vi "FPGAmain_5782_amtest.vi"() -> ()   [LabVIEW 2013]
uses:
  FPGA/DataMode.ctl
  FPGA/Input_5782/5782_states.ctl
  <vilib>/Platform/TimedLoop/XDataNode/timing_clust.ctl
  <vilib>/Platform/TimedLoop/XDataNode/nitl_modes.ctl
  <vilib>/Platform/TimedLoop/XDataNode/wakeup.ctl
  <vilib>/rvi/Emulation/niFpgaSctlEmulationGetInTimedLoop.vi
  <vilib>/rvi/Emulation/niFpgaEmulationReportErrorSimple.vi
  <vilib>/rvi/Emulation/niFpgaGetClockAttributes.vi
  <vilib>/rvi/eio/common/nirviEmuTemplateMethod_errors.vi
  <vilib>/rvi/Emulation/niFpgaCriticalErrorInLSC.vi
  <vilib>/rvi/FIFO/Fifo_Resource/nirvififoEmulationReadFpgaImpl.vi
  <vilib>/rvi/DataTransferAndStorage/Container/Common/niFpgaContainerGetUniqueNameForEmu.vi
  <vilib>/rvi/interface/RandomDataEmulation/nirviRandomDataFPGAFIFO.vi
  <vilib>/rvi/interface/RandomDataEmulation/niFpgaRandomDataHandleErrors.vi
  <vilib>/rvi/DataTransferAndStorage/Register/Emulation/niFpgaRegisterEmulationFpgaImpl.vi
  <instcachedir>/0/niFpgaRegisterEmulationFpgaImpl_DCF4BC0110594B98B44A971D60CEEC4D.lvgen/niFpgaRegisterEmulationFpgaImpl_DCF4BC0110594B98B44A971D60CEEC4D_003.vi
  <vilib>/rvi/FIFO/Fifo_Resource/nirvififoEmulationWriteFpgaImpl.vi
  <vilib>/Platform/TimedLoop/XDataNode/XDataNode.xnode
  <vilib>/eio/EIONode/EIONode.xnode
  <vilib>/rvi/DataTransferAndStorage/Container/XNode/niFpgaContainer.xnode
  <vilib>/rvi/FIFO/Fifo_Resource/nirvififoEmulationRead.vi
  <vilib>/rvi/interface/RandomDataEmulation/nirviRandomDataFpgaReadWriteTemplate.vi
  <vilib>/rvi/DataTransferAndStorage/Register/Emulation/niFpgaRegisterEmulation.vi
  <vilib>/rvi/FIFO/Fifo_Resource/nirvififoEmulationWrite.vi
  <vilib>/Platform/TimedLoop/XDataNode/XDNodeRunTimeDep.lvlib
panel:
  in  "b_am":fxp<+/-,16,2>
  in  "a_am":fxp<+/-,16,2>
  in  "AM phase":fxp<+,64,64>
  in  "DC offset chan 0":fxp<+/-,16,16>
  in  "DC offset chan 1":fxp<+/-,16,16>
  in  "delay phase":fxp<+,64,64>
  in  "User Command Commit":bool
  in  "User Command":u8
  out "User Command Idle":bool
  out "User Command Status":u8
  in  "User Data 0":u8
  in  "User Data 1":u8
  out "PLL Locked":bool
  out "User Error":bool
  out "Configured?":bool
  in  "Continuous":bool
  in  "trigger samples":u16=1
  in  "5782 record length":u16=4000 caption="Samples Per Trigger" min=1 step=1
  in  "Trigger Acquisition":bool
  out "IO Module\\Trigger Input":bool
  in  "quiet time":u16=4000
  in  "Downsample":fxp<+,8,8>=1.0
  in  "enable filter":bool
  in  "new coeffs":bool
  in  "FIR shift":i32
  in  "FIR coeffs":fxp<+/-,18,18>[](array[numeric])
  in  "Set downsample":bool
  in  "CIC Gain":fxp<+/-,32,1>=0.00390625 format="%#_32g"
  in  "Acquisition running":bool
  in  "Phase output":fxp<+,64,64>[](array[numeric])=[0.0, 0.0, 0.0, 0.0]
  in  "Simulated phase 5782":fxp<+,64,64>[](array[numeric])=[0.0, 0.0]
  in  "Mode":T1
  in  "Phase 5782":fxp<+,64,64>[](array[numeric])=[0.0, 0.0]
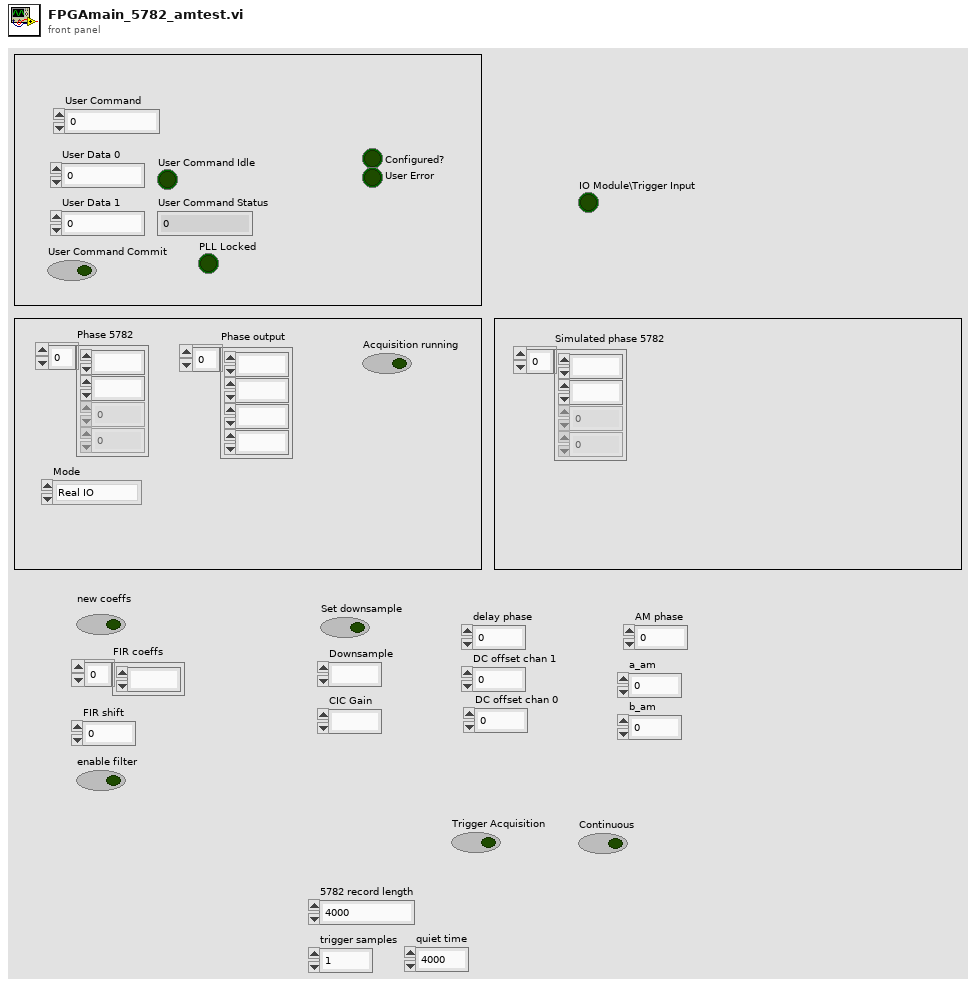
[diagram p1: front panel]
types:
  T1 = typedef "DataMode.ctl" = enum16{"Real IO", "Simulated"}
  T2 = typedef "5782_states.ctl" = enum8{"Wait for trigger", "Acquisition", "Send record length", "Quiet period"}
  T3 = typedef "XDNodeRunTimeDep.lvlib/timing_clust.ctl" = cluster{"Expected End [f-1]":u64, "Actual End [f-1]":u64, "Finished Late? [f-1]":bool, "Expected End [i-1]":u64, "Actual End [i-1]":u64, "Finished Late? [i-1]":bool, "Expected Start [i]":u64, "Actual Start [i]":u64, "Expected Start [f]":u64, "Actual Start [f]":u64, "Source Name":string, "Structure Name":string, "Period":i64, "Deadline":i64, "Offset":i64, "Start":i64, "Priority":i32, "Timeout":i32, "Mode":T4, "Wakeup Reason":T5, "Error":errorcluster, "Source Type":string, "Secondary Source Type":string, "Global End Time":u64, "Global Start Time":u64, "Frame Duration":u64, "Iteration Duration":u64, "Assigned CPU":i32, "I/O Scan Engine Mode":u32}
  T4 = typedef "XDNodeRunTimeDep.lvlib/nitl_modes.ctl" = enum32{"No Change", "Process missed periods, maintain original phase", "Discard missed periods, maintain original phase", "Process missed periods, ignore original phase", "Discard missed periods, ignore original phase"}
  T5 = typedef "XDNodeRunTimeDep.lvlib/wakeup.ctl" = enum32{"Normal", "Aborted", "Asynchronous wakeup", "Timing source error", "Timed loop error", "Timeout"}
  T6 = typedef "I16 array size 2.ctl" = i16[]
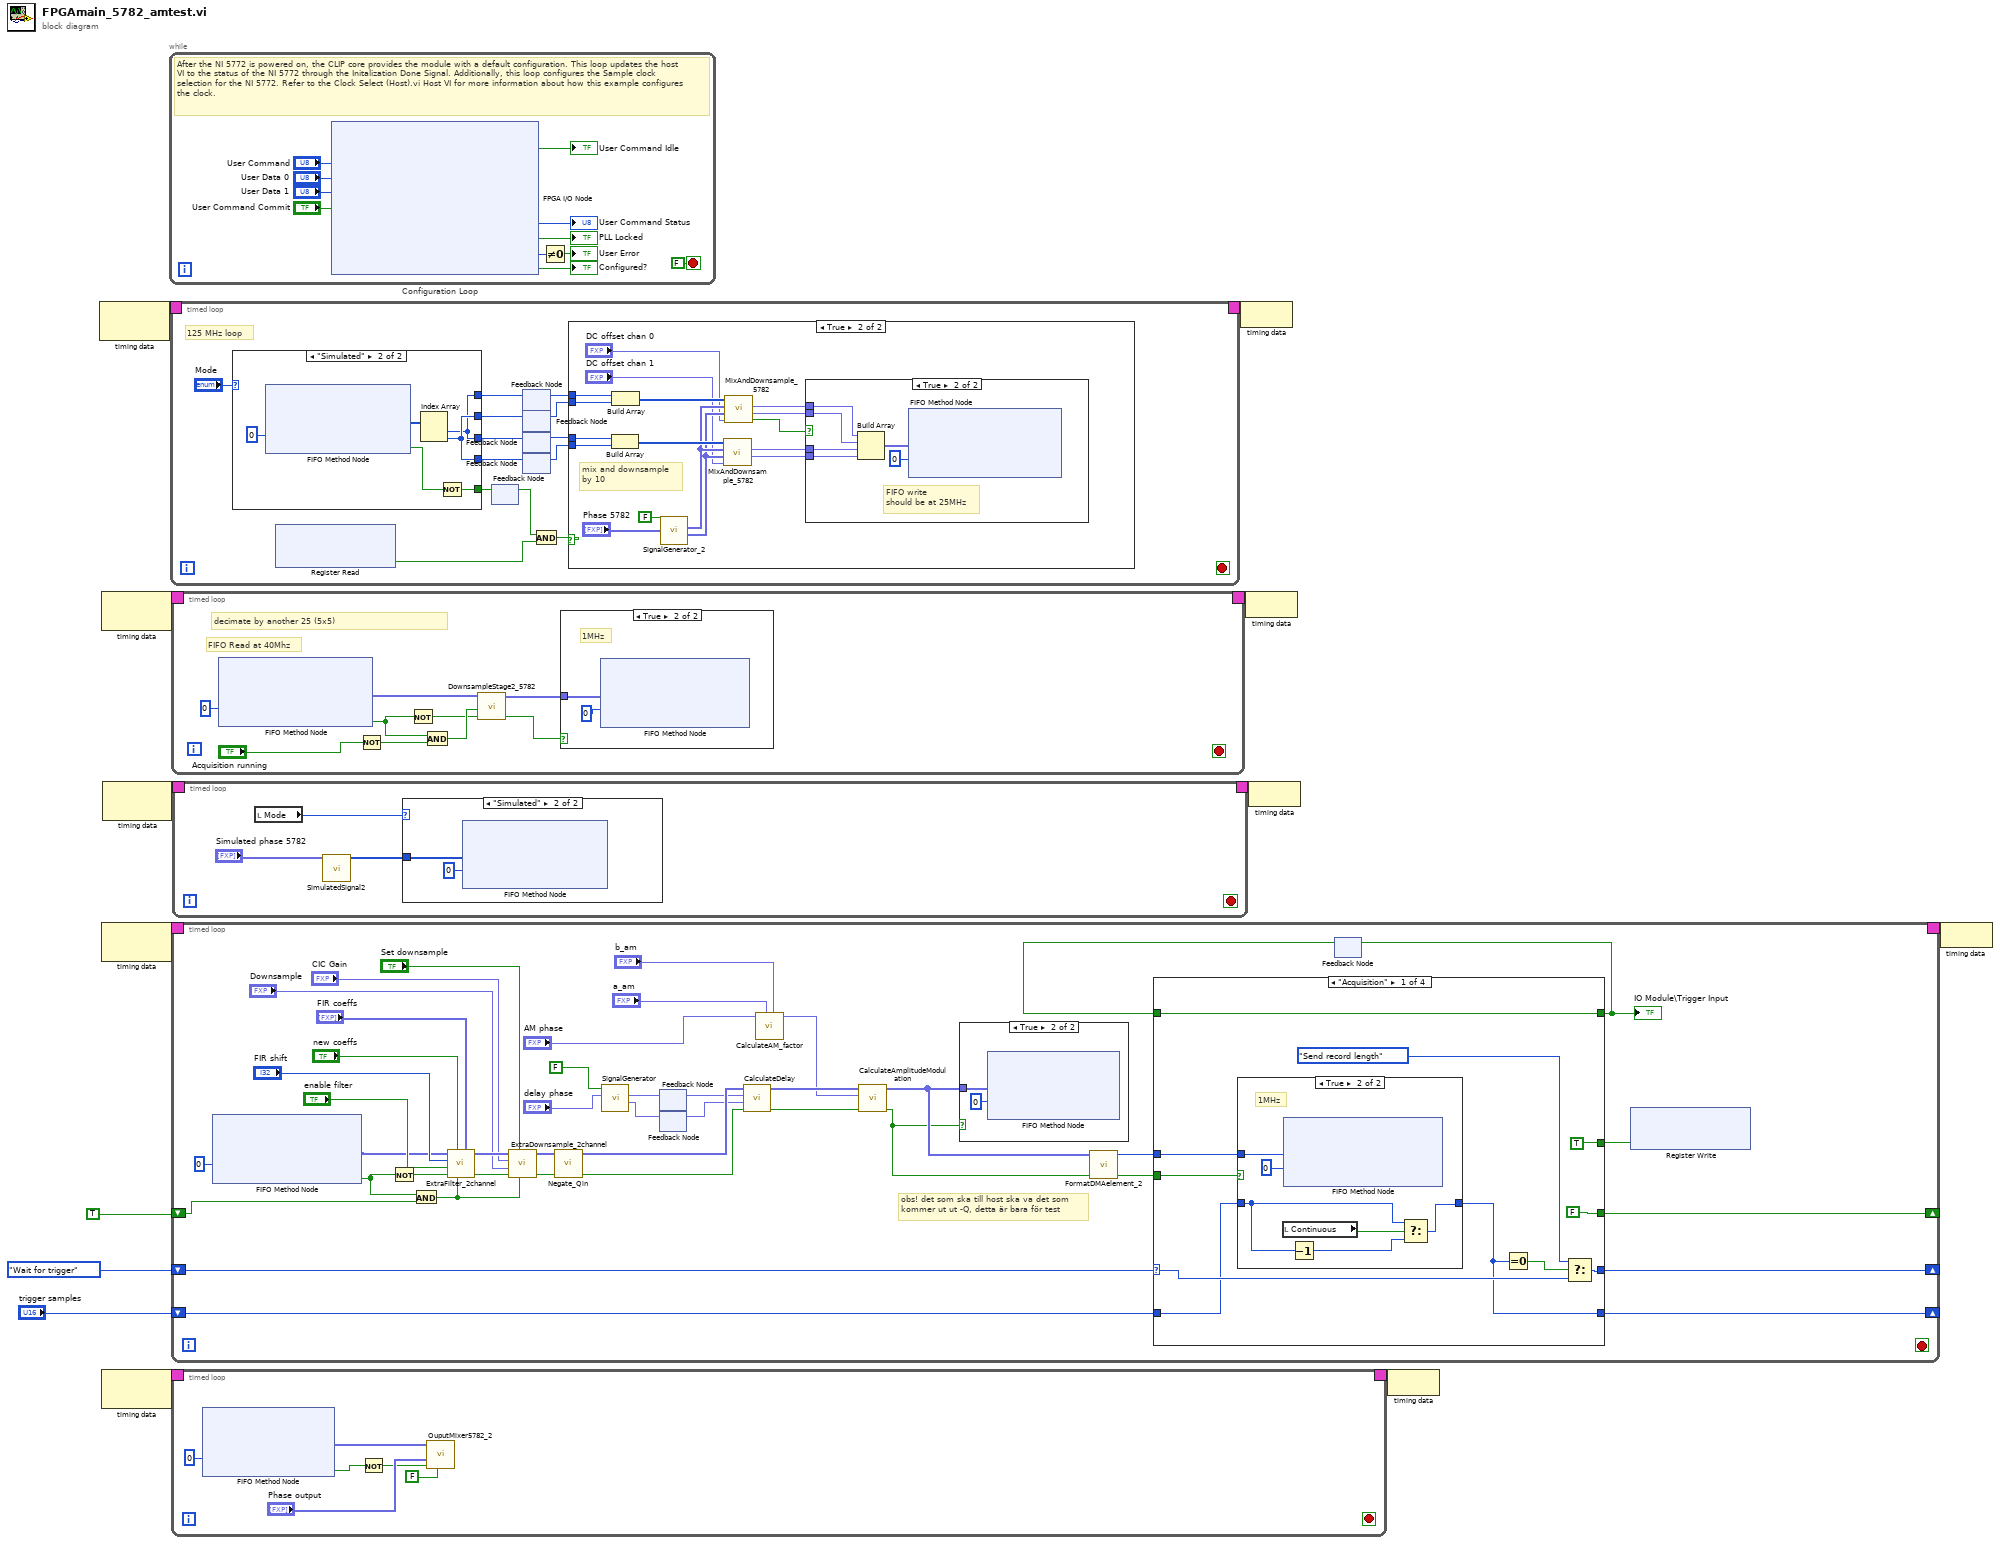
[diagram p0: block diagram]
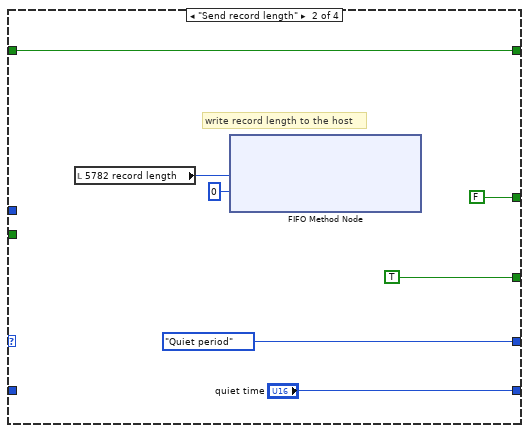
[diagram p4: hidden frame]
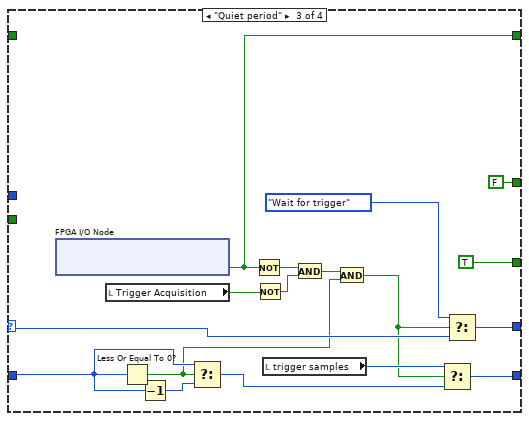
[diagram p5: hidden frame]
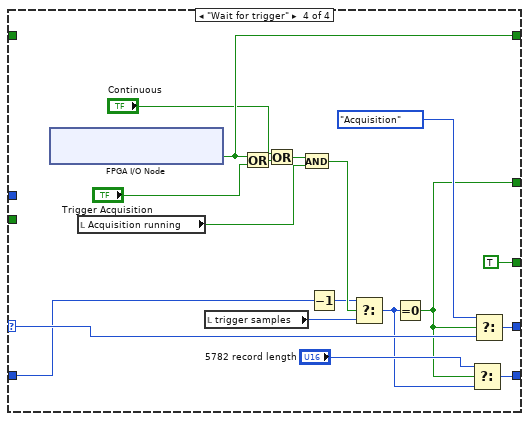
[diagram p6: hidden frame]
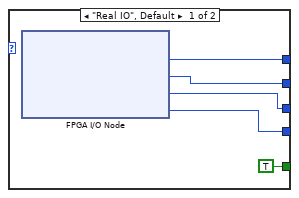
[diagram p9: hidden frame]
diagram:
  n1 = node-c288() -> (w9:T3)  [unwired: 1 in]
  n2 = node-c288() -> (w13:T3)  [unwired: 1 in]
  n3 = node-c288() -> (w7:T3)  [unwired: 1 in]
  n4 = node-c288() -> (w2:T3)  [unwired: 1 in]
  n5 = node-c288() -> (w11:T3)  [unwired: 1 in]
  n6 = while "Configuration Loop" {
    stop <- FALSE stop-if-true
    # "After the NI 5772 is powered on, the CLIP core provides the module with a default configuration. This loop updates the host VI to the status of the NI 5772 through the Initalization Done Signal. Additionally, this loop configures the Sample clock selection for the NI 5772. Refer to the Clock Select (Host).vi Host VI for more information about how this example configures the clock."
    n7 = xnode "FPGA I/O Node"("IO Module\\User Command"="User Command", "IO Module\\User Data 0"="User Data 0", "IO Module\\User Data 1"="User Data 1", "IO Module\\User Command Commit"="User Command Commit") -> ("IO Module\\User Command Idle"=→"User Command Idle":bool, "IO Module\\User Command Status"=→"User Command Status":u8, "IO Module\\PLL Locked"=→"PLL Locked":bool, "IO Module\\User Error"=w19:u8, "IO Module\\Initialization Done"=→"Configured?":bool)  [unwired: 9 in, 9 out]
    n8 = Not Equal To 0?(x=w19) -> (x != 0?=→"User Error":bool)
  }
  n9 = timed-loop {
    timing: w9 -> [_]
    timing-out: [_] -> w8
    stop <- _ stop-if-true
    # "125 MHz loop"
    n10 = case shown="\"Simulated\"" "Mode" {
      tunnel: [w65 w68] -> w35
      tunnel: [w64 w69] -> w33
      tunnel: [w63 w68] -> w31
      tunnel: [w62 w69] -> w28
      tunnel: [TRUE w66] -> w27
      frame "Real IO", Default {
        n11 = xnode "FPGA I/O Node"() -> ("IO Module\\AI 0 N-1"=w65:i16, "IO Module\\AI 0 N"=w64:i16, "IO Module\\AI 1 N-1"=w63:i16, "IO Module\\AI 1 N"=w62:i16)  [unwired: 4 in, 4 out]
      }
      frame "Simulated" {
        n12 = xnode ("FIFO Method Node")("Timeout"=0) -> ("Element"=w70:i16[], "Timed Out?"=w67:bool)  [unwired: 1 in, 1 out]
        n13 = Index Array(array=w70) -> (element #1=w68:i16, element #2=w69:i16)  [unwired: 2 in]
        n14 = Not(x=w67) -> (.not. x?=w66:bool)
      }
    }
    n15 = xnode ("Register Read")() -> ("Data"=w25:bool)  [unwired: 1 in, 1 out]
    n16 = feedback #1() -> (w26:bool)  [unwired: 1 in]
    n17 = feedback-in #1(w27) -> ()
    n18 = feedback #2() -> (w34:i16)  [unwired: 1 in]
    n19 = feedback-in #2(w35) -> ()
    n20 = feedback #3() -> (w32:i16)  [unwired: 1 in]
    n21 = feedback-in #3(w33) -> ()
    n22 = feedback #4() -> (w30:i16)  [unwired: 1 in]
    n23 = feedback-in #4(w31) -> ()
    n24 = feedback #5() -> (w29:i16)  [unwired: 1 in]
    n25 = feedback-in #5(w28) -> ()
    n26 = And(x=w26, y=w25) -> (x .and. y?=w36:bool)
    n27 = case shown="True" w36 {
      tunnel: w34 -> [_ w45]
      tunnel: w32 -> [_ w44]
      tunnel: w30 -> [_ w43]
      tunnel: w29 -> [_ w42]
      frame False {
      }
      frame True {
        # "mix and downsample\nby 10"
        n28 = Build Array(w43, w42) -> (w54:i16[])
        n29 = Build Array(w45, w44) -> (w41:i16[])
        n30 = call "SignalGenerator_2.vi"("Phase"="Phase 5782", "reset"=FALSE) -> ("Sine out"=w46:fxp<+/-,16,0>[], "Cosine out"=w47:fxp<+/-,16,0>[])  [unwired: 8 in]
        n31 = call "MixAndDownsample_5782.vi"("DC offset"="DC offset chan 1", "Sine in"=w46, "Cosine in"=w47, "Signal Input"=w54) -> ("Q out"=w49:fxp<+/-,16,14>, "I out"=w50:fxp<+/-,16,14>)  [unwired: 5 in, 1 out]
        n32 = call "MixAndDownsample_5782.vi"("DC offset"="DC offset chan 0", "Sine in"=w46, "Cosine in"=w47, "Signal Input"=w41) -> ("data valid"=w51:bool, "Q out"=w52:fxp<+/-,16,14>, "I out"=w53:fxp<+/-,16,14>)  [unwired: 5 in]
        n33 = case shown="True" w51 {
          tunnel: w52 -> [_ w60]
          tunnel: w53 -> [_ w57]
          tunnel: w50 -> [_ w56]
          tunnel: w49 -> [_ w55]
          frame False {
          }
          frame True {
            # "FIFO write\nshould be at 25MHz"
            n34 = Build Array(w57, w60, w56, w55) -> (w59:fxp<+/-,16,14>[])
            n35 = xnode ("FIFO Method Node")("Element"=w59, "Timeout"=0) -> ()  [unwired: 1 in, 2 out]
          }
        }
      }
    }
  }
  n36 = timed-loop {
    timing: w13 -> [_]
    timing-out: [_] -> w12
    stop <- _ stop-if-true
    # "FIFO Read at 40Mhz"
    # "decimate by another 25 (5x5)"
    n37 = xnode ("FIFO Method Node")("Timeout"=0) -> ("Element"=w81:fxp<+/-,16,14>[], "Timed Out?"=w77:bool)  [unwired: 1 in, 1 out]
    n38 = Not(x="Acquisition running") -> (.not. x?=w78:bool)
    n39 = Not(x=w77) -> (.not. x?=w75:bool)
    n40 = And(x=w77, y=w78) -> (x .and. y?=w76:bool)
    n41 = call "DownsampleStage2_5782.vi"("valid in"=w75, "reset"=w76, "Data in"=w81) -> ("valid out"=w79:bool, "data out"=w80:fxp<+/-,16,14>[])  [unwired: 7 in]
    n42 = case shown="True" w79 {
      tunnel: w80 -> [_ w83]
      frame False {
      }
      frame True {
        # "1MHz"
        n43 = xnode ("FIFO Method Node")("Element"=w83, "Timeout"=0) -> ()  [unwired: 1 in, 2 out]
      }
    }
  }
  n44 = timed-loop {
    timing: w7 -> [_]
    timing-out: [_] -> w6
    shift-right: [w127] -> _
    shift-left: 5782_states."Wait for trigger" ("5782 states") -> [w129]
    shift-right: [w126] -> _
    shift-left: "trigger samples" -> [w128]
    shift-right: [w108] -> _
    shift-left: TRUE -> [w111]
    stop <- _ stop-if-true
    # "obs! det som ska till host ska va det som\nkommer ut ut -Q, detta är bara för test"
    n45 = xnode ("FIFO Method Node")("Timeout"=0) -> ("Element"=w113:fxp<+/-,16,14>[], "Timed Out?"=w112:bool)  [unwired: 1 in, 1 out]
    n46 = Not(x=w112) -> (.not. x?=w122:bool)
    n47 = And(x=w112, y=w111) -> (x .and. y?=w124:bool)
    n48 = call "ExtraFilter_2channel.vi"(5:"new coeffs"="FIR coeffs", "reset"=w124, 7:"new coeffs"="new coeffs", "valid in"=w122, "enable filter"="enable filter", "new shift"="FIR shift", "Data in"=w113) -> ("valid out"=w123:bool, "Data out"=w121:fxp<+/-,16,14>[])  [unwired: 3 in]
    n49 = call "ExtraDownsample_2channel.vi"("reset"=w124, "Set downsample"="Set downsample", "valid in"=w123, "Downsample"="Downsample", "CIC Gain"="CIC Gain", "Data in"=w121) -> ("valid out"=w103:bool, "Data out"=w104:fxp<+/-,16,14>[])  [unwired: 4 in]
    n50 = call "Negate_Qin.vi"("valid in"=w103, "Data in"=w104) -> ("valid out"=w102:bool, "Data out"=w101:fxp<+/-,16,14>[])  [unwired: 8 in]
    n51 = call "SignalGenerator.vi"("phase"="delay phase", "Reset"=FALSE) -> ("Cos"=w97:fxp<+/-,16,0>, "Sin"=w98:fxp<+/-,16,0>)  [unwired: 7 in, 1 out]
    n52 = feedback-in #6(w98) -> ()
    n53 = feedback #6() -> (w96:fxp<+/-,16,0>)  [unwired: 1 in]
    n54 = feedback #7() -> (w95:fxp<+/-,16,0>)  [unwired: 1 in]
    n55 = feedback-in #7(w97) -> ()
    n56 = call "CalculateDelay.vi"("input valid"=w102, "cos_fi"=w95, "sin fi"=w96, "Data in"=w101) -> ("output valid"=w93:bool, "Data out"=w94:fxp<+/-,16,14>[])  [unwired: 6 in]
    n57 = call "CalculateAM_factor.vi"("b_am"="b_am", "a_am"="a_am", "AM phase"="AM phase") -> ("AM_factor"=w87:fxp<+/-,16,2>)  [unwired: 7 in, 1 out]
    n58 = call "CalculateAmplitudeModulation.vi"("input valid"=w93, "AM_factor"=w87, "Data in"=w94) -> ("output valid"=w91:bool, "Data out"=w92:fxp<+/-,16,14>[])  [unwired: 7 in]
    n59 = case shown="True" w91 {
      tunnel: w92 -> [_ w130]
      frame False {
      }
      frame True {
        n60 = xnode ("FIFO Method Node")("Element"=w130, "Timeout"=0) -> ()  [unwired: 1 in, 2 out]
      }
    }
    n61 = call "FormatDMAelement_2.vi"("valid in"=w91, "Data in"=w92) -> ("valid out"=w109:bool, "Element1"=w110:u64)  [unwired: 8 in]
    n62 = feedback #8() -> (w106:bool)  [unwired: 1 in]
    n63 = case shown="\"Acquisition\"" w129 {
      selector: w129 -> [w142 _ w171 w191]
      tunnel: w128 -> [w138 _ w159 w178]
      tunnel: [w141 5782_states."Quiet period" ("5782 states") w170 w190] -> w127
      tunnel: [w135 "quiet time" w173 w189] -> w126
      tunnel: w110 -> [w136 _ _ _]
      tunnel: w109 -> [w137 _ _ _]
      tunnel: [FALSE TRUE TRUE TRUE] -> w108
      tunnel: [TRUE FALSE ("5782 triggered") FALSE ("5782 triggered") w182] -> w107
      tunnel: [w134 w150 w161 w181] -> w105
      tunnel: w106 -> [w134 w150 _ _]
      frame "Acquisition" {
        n64 = case shown="True" w137 {
          tunnel: w136 -> [_ w149]
          tunnel: [w143 w146] -> w135
          tunnel: w138 -> [w143 w144]
          frame False {
          }
          frame True {
            # "1MHz"
            n65 = local read "Continuous"() -> (w147:bool)
            n66 = xnode ("FIFO Method Node")("Element"=w149, "Timeout"=0) -> ()  [unwired: 1 in, 2 out]
            n67 = Decrement(x=w144) -> (x-1=w145:u16)
            n68 = Select(t=w144, s=w147, f=w145) -> (s? t:f=w146:u16)
          }
        }
        n69 = Equal To 0?(x=w135) -> (x = 0?=w139:bool)
        n70 = Select(t=5782_states."Send record length" ("5782 states"), s=w139, f=w142) -> (s? t:f=w141:T2)
      }
      frame "Send record length" {
        # "write record length to the host"
        n71 = local read "5782 record length"() -> (w152:u16)
        n72 = xnode ("FIFO Method Node")("Element"=w152, "Timeout"=0) -> ()  [unwired: 1 in, 2 out]
      }
      frame "Quiet period" {
        n73 = xnode "FPGA I/O Node"() -> ("IO Module\\Trigger Input"=w161:bool)  [unwired: 1 in, 1 out]
        n74 = local read "Trigger Acquisition"() -> (w167:bool)
        n75 = Less Or Equal To 0?(x=w159) -> (x <= 0?=w158:bool)
        n76 = Decrement(x=w159) -> (x-1=w160:u16)
        n77 = Select(t=w159, s=w158, f=w160) -> (s? t:f=w157:u16)
        n78 = Not(x=w161) -> (.not. x?=w166:bool)
        n79 = Not(x=w167) -> (.not. x?=w165:bool)
        n80 = local read "trigger samples"() -> (w172:u16)
        n81 = And(x=w166, y=w165) -> (x .and. y?=w164:bool)
        n82 = And(x=w164, y=w158) -> (x .and. y?=w169:bool)
        n83 = Select(t=w172, s=w169, f=w157) -> (s? t:f=w173:u16)
        n84 = Select(t=5782_states."Wait for trigger" ("5782 states"), s=w169, f=w171) -> (s? t:f=w170:T2)
      }
      frame "Wait for trigger" {
        n85 = xnode "FPGA I/O Node"() -> ("IO Module\\Trigger Input"=w181:bool)  [unwired: 1 in, 1 out]
        n86 = local read "Acquisition running"() -> (w183:bool)
        n87 = local read "trigger samples"() -> (w177:u16)
        n88 = Or(x=w181, y="Trigger Acquisition") -> (x .or. y?=w176:bool)
        n89 = Or(x="Continuous", y=w176) -> (x .or. y?=w174:bool)
        n90 = And(x=w174, y=w183) -> (x .and. y?=w184:bool)
        n91 = Decrement(x=w178) -> (x-1=w179:u16)
        n92 = Select(t=w179, s=w184, f=w177) -> (s? t:f=w180:u16)
        n93 = Equal To 0?(x=w180) -> (x = 0?=w182:bool)
        n94 = Select(t="5782 record length", s=w182, f=w180) -> (s? t:f=w189:u16)
        n95 = Select(t=5782_states."Acquisition" ("5782 states"), s=w182, f=w191) -> (s? t:f=w190:T2)
      }
    }
    "IO Module\\Trigger Input" <- w105
    n96 = feedback-in #8(w105) -> ()
    n97 = xnode ("Register Write")("Data"=w107) -> ()  [unwired: 1 in, 1 out]
  }
  n98 = timed-loop {
    timing: w2 -> [_]
    timing-out: [_] -> w1
    stop <- _ stop-if-true
    n99 = xnode ("FIFO Method Node")("Timeout"=0) -> ("Element"=w196:fxp<+/-,16,14>[], "Timed Out?"=w198:bool)  [unwired: 1 in, 1 out]
    n100 = Not(x=w198) -> (.not. x?=w194:bool)
    n101 = call "OuputMixer5782_2.vi"("reset"=FALSE, "valid in"=w194, "Phase output"="Phase output", "Data in"=w196) -> ()  [unwired: 7 in, 1 out]
  }
  n102 = timed-loop {
    timing: w11 -> [_]
    timing-out: [_] -> w10
    stop <- _ stop-if-true
    n103 = local read "Mode"() -> (w204:T1)
    n104 = call "SimulatedSignal2.vi"("Phase"="Simulated phase 5782") -> ("output"=w203:T6)  [unwired: 9 in, 1 out]
    n105 = case shown="\"Simulated\"" w204 {
      tunnel: w203 -> [_ w205]
      frame "Real IO", Default {
      }
      frame "Simulated" {
        n106 = xnode ("FIFO Method Node")("Element"=w205, "Timeout"=0) -> ()  [unwired: 1 in, 2 out]
      }
    }
  }
  n107 = node-c288(w8) -> ()
  n108 = node-c288(w12) -> ()
  n109 = node-c288(w10) -> ()
  n110 = node-c288(w1) -> ()
  n111 = node-c288(w6) -> ()
